vi "MPB Sequences.vi"(8 "error in":errorcluster, 9 "Tag Name":string, 10 "sequence number":i32) -> (0 "error out":errorcluster, 2 "(description) used in test":string)   [LabVIEW 2020]
uses:
  Ethernet_IP/EIP.ctl
  <vilib>/AKKA/PROVEtech-RBS/PROVEtechRBS.lvlib
  <vilib>/AKKA/PROVEtech-RBS/SubVIs/Read (Signals Single-point).vi
  <vilib>/AKKA/PROVEtech-RBS/SubVIs/Write (Signals Single-point).vi
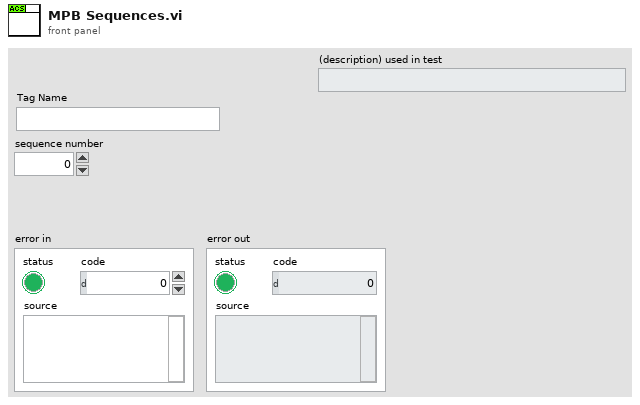
[diagram p1: front panel]
types:
  T1 = typedef "EIP.ctl" = enum16{"Open", "Close", "Tag Read SINT", "Tag Read INT", "Tag Read DINT", "Tag Read REAL", "Tag Read BOOL", "Tag Read STRING", "Tag Read RAW", "Tag Write SINT", "Tag Write INT", "Tag Write DINT", "Tag Write REAL", "Tag Write BOOL", "Tag Write STRING", "Tag Write Raw"}
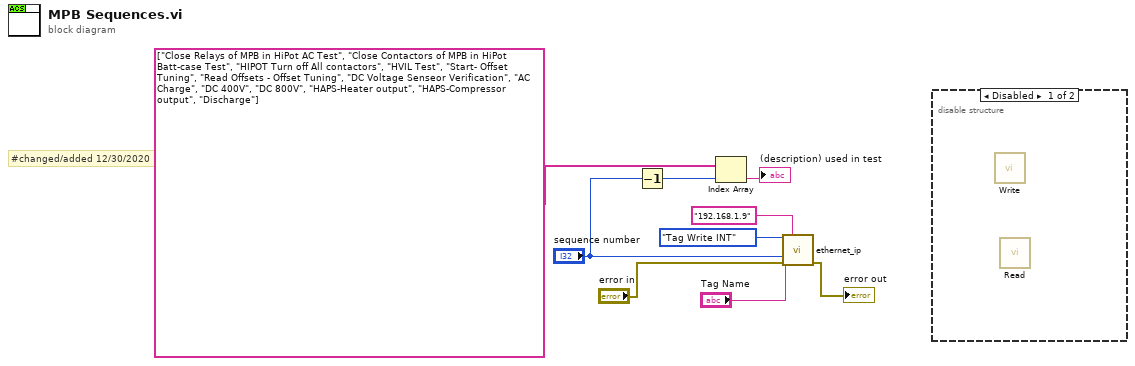
[diagram p0: block diagram]
diagram:
  # "#changed/added 12/30/2020"
  n1 = Decrement(x="sequence number") -> (x-1=w8:i32)
  n2 = Index Array(array=string[] ["Close Relays of MPB in HiPot AC Test", "Close Contactors of MPB in HiPot Batt-case Test", "HIPOT Turn off All contactors", "HVIL Test", "Start- Offset Tuning", "Read Offsets - Offset Tuning", "DC Voltage Senseor Verification", "AC Charge", "DC 400V", "DC 800V", "HAPS-Heater output", "HAPS-Compressor output", "Discharge"], index=w8) -> (element=→"(description) used in test":string)
  n3 = call "ethernet_ip.vi"("EIP"=EIP."Tag Write INT", "network path"="192.168.1.9", "Tag Name"="Tag Name", "data in"="sequence number", "error in (no error)"="error in") -> ("error out"=→"error out":errorcluster)  [unwired: 2 in, 8 out]
  n4 = disable-structure shown="Disabled" {
    frame Disabled {
      n5 = call-poly <vilib>:"Write.vi"() -> ()  [unwired: 10 in, 2 out]
      n6 = call-poly <vilib>:"Read.vi"() -> ()  [unwired: 9 in, 3 out]
    }
    frame Enabled {
    }
  }
